vi "Handle low Press.vi"(8 "error in (no error)":errorcluster, 11 "Stand in":refnum<class "Stand.lvclass">) -> (0 "error out":errorcluster, 3 "Stand out":refnum<class "Stand.lvclass">)   [LabVIEW 2019, in "Stand.lvclass"]
uses:
  Stand.lvclass
  D:/GIT H4000/H4000/src/Device_class/Device.lvclass
  Stand.lvclass/Stand.ctl
  TypeDef/handleModeState.ctl
  Device_class/Device.lvclass/Device.ctl
  FPGA/TypeDef/DO index.ctl
  TypeDef/Active Motor.ctl
  TypeDef/Motor N.ctl
  AI_class/AI.lvclass/AI.ctl
  AnalogComparator_class/AnalogComparator.lvclass/AnalogComparator.ctl
  OscillationClass/OscillationDetector.lvclass/OscillationDetector.ctl
  AI_class/Get_Values.vi
  AnalogComparator_class/GetStatus.vi
  OscillationClass/Read DATA.vi
  FPGA_API_class/FPGA API.lvclass
  Device_class/Device.lvclass
  PM_Group_class/PM_Group.lvclass
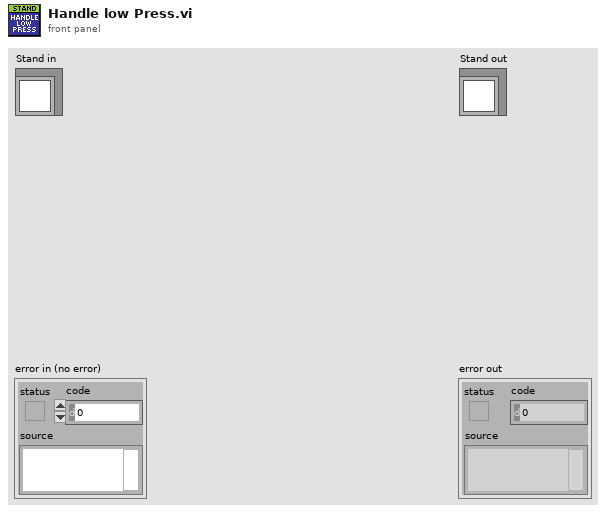
[diagram p1: front panel]
types:
  T1 = typedef "Step_Name.ctl" = enum16{"IDLE", "Filling", "Low Pressure", "Hi Pressure", "Abrupt Pressure Release", "Smooth Pressure Release", "Measuring Leakage Sensor 41.3", "Measuring Leakage Burette 42", "Alarm", "Stop Pump"}
  T2 = typedef "handleModeState.ctl" = enum16{"Init", "Run"}
  T3 = typedef "Active Motor.ctl" = cluster{"Active":bool, "MotorN":T4}
  T4 = typedef "Motor N.ctl" = enum16{"M12", "M21", "M24"}
  T5 = typedef "Direction.ctl" = enum16{"None", "DUT", "Chamber"}
  T6 = typedef "DO index.ctl" = u8
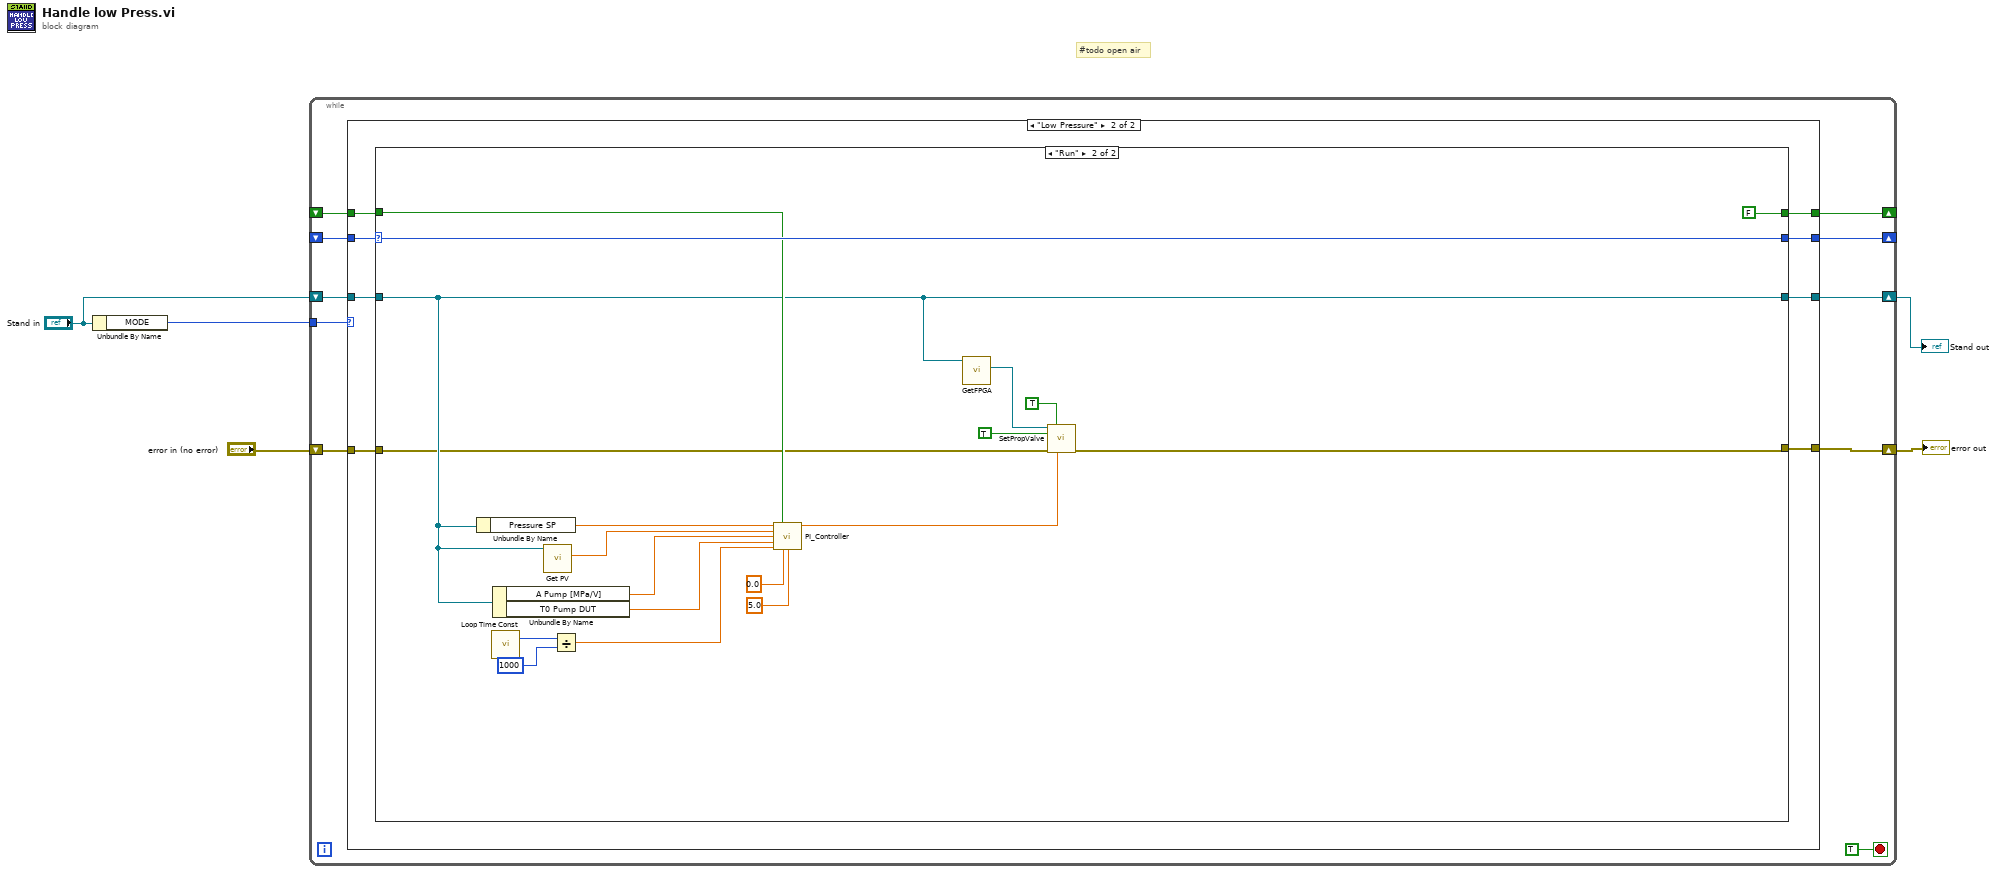
[diagram p0: block diagram]
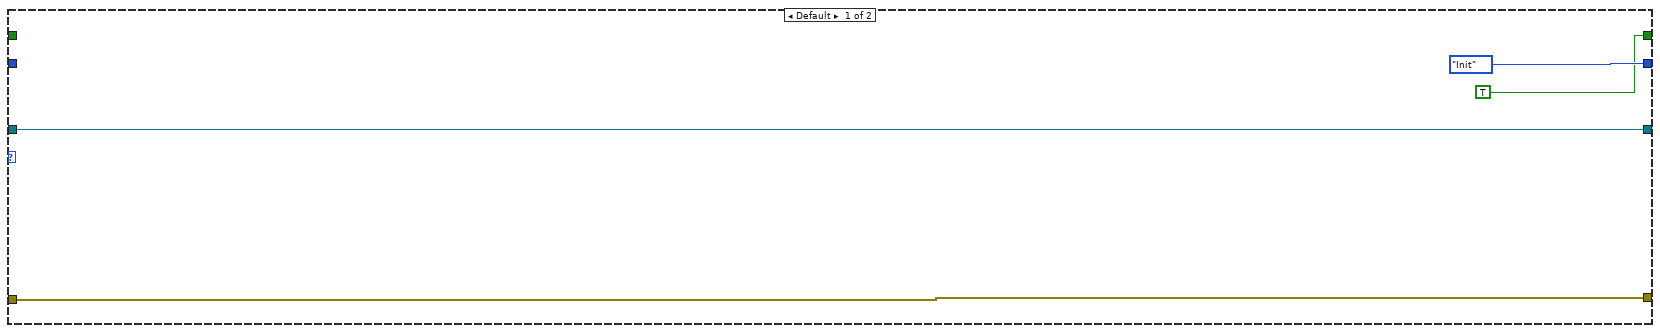
[diagram p2: hidden frame]
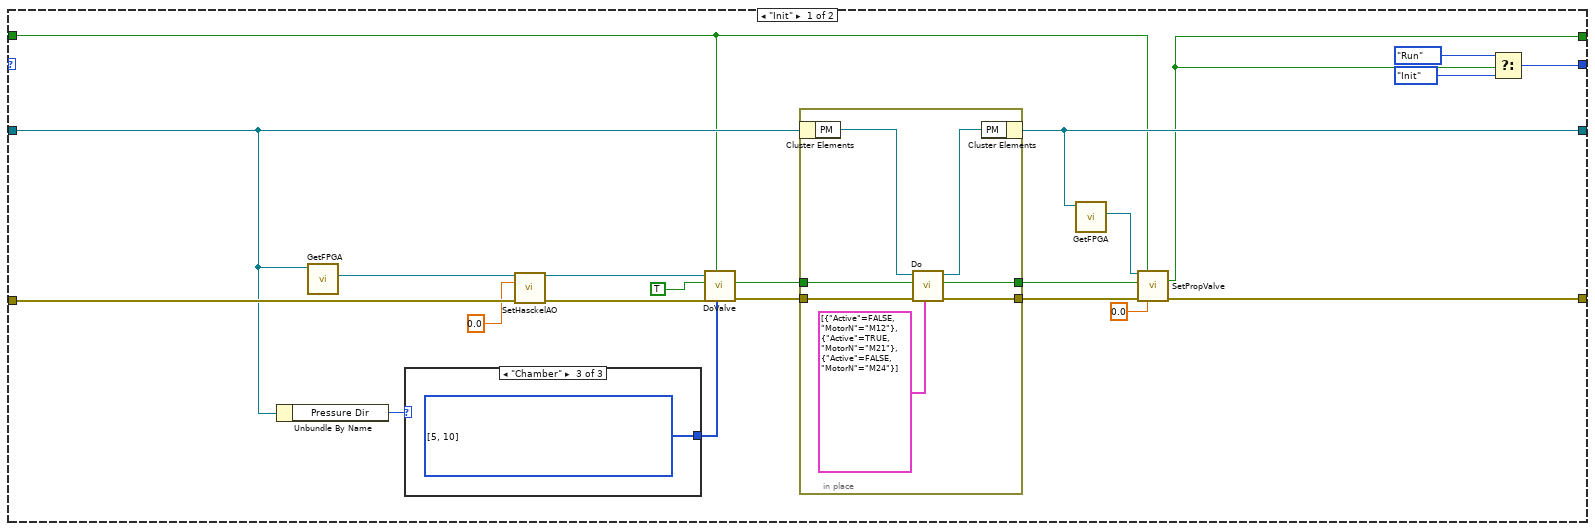
[diagram p3: hidden frame]
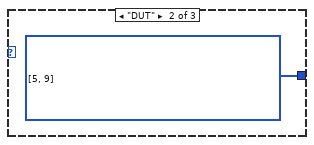
[diagram p5: hidden frame]
diagram:
  # "#todo open air"
  n1 = Unbundle By Name("Stand in") -> ("MODE"=w2:T1)
  n2 = while {
    tunnel: w2 -> [w12]
    shift-right: [w15] -> w5
    shift-left: "error in (no error)" -> [w14]
    shift-right: [w11] -> w1
    shift-left: "Stand in" -> [w13]
    shift-right: [w9] -> _
    shift-left: _ -> [w8]
    shift-right: [w7] -> _
    shift-left: _ -> [w6]
    stop <- TRUE stop-if-true
    n3 = case shown="\"Low Pressure\"" w12 {
      tunnel: w14 -> [w19 w26]
      tunnel: [w19 w27] -> w15
      tunnel: w13 -> [w18 w25]
      tunnel: [w18 w24] -> w11
      tunnel: [handleModeState."Init" ("handleModeState") w20] -> w9
      tunnel: w8 -> [_ w23]
      tunnel: [TRUE w21] -> w7
      tunnel: w6 -> [_ w22]
      frame Default {
      }
      frame "Low Pressure" {
        n4 = case shown="\"Run\"" w23 {
          selector: w23 -> [_ w77]
          tunnel: [w42 w59] -> w27
          tunnel: w26 -> [w49 w62]
          tunnel: w25 -> [w45 w64]
          tunnel: [w48 w64] -> w24
          tunnel: w22 -> [w44 w75]
          tunnel: [w28 FALSE] -> w21
          tunnel: [w47 w77] -> w20
          frame "Init" {
            n5 = Unbundle By Name(w45) -> ("Pressure Dir"=w39:T5)
            n6 = call "GetFPGA.vi"("Device in"=w45) -> ("FPGA API.lvclass"=w36:refnum<class "FPGA API.lvclass">)  [unwired: 10 in]
            n7 = case shown="\"Chamber\"" w39 {
              tunnel: [_ w50 w51] -> w38
              frame Default {
              }
              frame "DUT" {
                w50 = T6[] [5, 9] items=["DO 0 [KP1] [M12]", "DO 1 [ON KP2] [M21]", "DO 2 [ON KP3] [M24]", "DO 3 [WATER Y18.1 [DO3]]", "DO 4 [WATER Y18.2 [DO4]]", "DO 5 [KP6 Y29.1 33.7]", "DO 6 [KP7 Y29.2 33.8]", "DO 7 [KP8 Y29.3 33.9]", "DO 8 [KP9 Y29.4  33.12]", "DO 9 [KP10 Y29.5 33.1]", "DO 10 [KP11 Y29.6 33.2]", "DO 11 [KP12 Y29.7  33.13]", "DO 12 [KP13 Y29.8  33.11]", "DO 13 [KP14 Y29.9 33.10]", "DO 14 [KP15 Y29.10  33.6]", "DO 15 [KP16 Y29.11  33.5]", "DO 16 [KP17 Y29.12  33.4]", "DO 17 [KP18 Y29.13 33.3]", "DO 18 [AIR KP19]", "DO 19 [STEP DRIVE EN KP20]", "DO 20 [KP21 Y44.1 OPEN]", "DO 21 [ KP22 Y44.1 CLOSE]", "DO 22 [ KP23 Y44.2 OPEN]", "DO 23", "DO 24 [STEP DRIVE 1]", "DO 25 [STEP DRIVE 2]"] ("#DO")
              }
              frame "Chamber" {
                w51 = T6[] [5, 10] items=["DO 0 [KP1] [M12]", "DO 1 [ON KP2] [M21]", "DO 2 [ON KP3] [M24]", "DO 3 [WATER Y18.1 [DO3]]", "DO 4 [WATER Y18.2 [DO4]]", "DO 5 [KP6 Y29.1 33.7]", "DO 6 [KP7 Y29.2 33.8]", "DO 7 [KP8 Y29.3 33.9]", "DO 8 [KP9 Y29.4  33.12]", "DO 9 [KP10 Y29.5 33.1]", "DO 10 [KP11 Y29.6 33.2]", "DO 11 [KP12 Y29.7  33.13]", "DO 12 [KP13 Y29.8  33.11]", "DO 13 [KP14 Y29.9 33.10]", "DO 14 [KP15 Y29.10  33.6]", "DO 15 [KP16 Y29.11  33.5]", "DO 16 [KP17 Y29.12  33.4]", "DO 17 [KP18 Y29.13 33.3]", "DO 18 [AIR KP19]", "DO 19 [STEP DRIVE EN KP20]", "DO 20 [KP21 Y44.1 OPEN]", "DO 21 [ KP22 Y44.1 CLOSE]", "DO 22 [ KP23 Y44.2 OPEN]", "DO 23", "DO 24 [STEP DRIVE 1]", "DO 25 [STEP DRIVE 2]"] ("#DO")
              }
            }
            n8 = call-dynamic "SetHasckelAO.vi"("FPGA API in"=w36, "Haskel in"=0.0, "error in (no error)"=w49) -> ("FPGA API out"=w41:refnum<class "FPGA API.lvclass">, "error out"=w40:errorcluster)  [unwired: 11 in]
            n9 = call "DoValve.vi"("#DO"=w38, "Init"=w44, "error in (no error)"=w40, "Do"=TRUE, "reference in"=w41) -> ("error out"=w34:errorcluster, "Done"=w33:bool)  [unwired: 4 in, 1 out]
            n10 = in-place {
              in-place-border: w34 -> [w57]
              in-place-border: w33 -> [w55]
              in-place-border: [w54] -> w32
              in-place-border: [w53] -> w30
              n11 = in-place-cluster #1(w45) -> ("PM"=w58:refnum<class "PM_Group.lvclass">)
              n12 = call "Do.vi"("Data"=T3[] [{"Active"=FALSE, "MotorN"=enum."M12"}, {"Active"=TRUE, "MotorN"=enum."M21"}, {"Active"=FALSE, "MotorN"=enum."M24"}] ("Array"), "error in (no error)"=w57, "Do"=w55, "PM_Group in"=w58) -> ("error out"=w54:errorcluster, "Done"=w53:bool, "PM_Group out"=w56:refnum<class "PM_Group.lvclass">)  [unwired: 5 in]
              n13 = in-place-cluster #1("PM"=w56) -> (w48:refnum<class "Stand.lvclass">)
            }
            n14 = call "GetFPGA.vi"("Device in"=w48) -> ("FPGA API.lvclass"=w31:refnum<class "FPGA API.lvclass">)  [unwired: 10 in]
            n15 = call-dynamic "SetPropValve.vi"("FPGA API in"=w31, "Init"=w44, "Do"=w30, "error in (no error)"=w32, "AO 1"=0.0) -> ("Done"=w28:bool, "error out"=w42:errorcluster)  [unwired: 8 in, 1 out]
            n16 = Select(t=handleModeState."Run", s=w28, f=handleModeState."Init") -> (s? t:f=w47:T2)
          }
          frame "Run" {
            n17 = Unbundle By Name(w64) -> ("Pressure SP"=w74:dbl)
            n18 = call "Loop Time Const.vi"() -> ("loop time ms"=w68:i64)  [unwired: 3 in]
            n19 = Unbundle By Name(w64) -> ("A Pump [MPa/V]"=w72:dbl, "T0 Pump DUT"=w69:dbl)
            n20 = call "Get PV.vi"("Stand in"=w64) -> ("Stat Data.scl mean"=w73:dbl)  [unwired: 10 in]
            n21 = Divide(x=w68, y=i64 1000) -> (x/y=w66:dbl)
            n22 = call "PI_Controller.vi"("SP"=w74, "Init"=w75, "PV"=w73, "A"=w72, "T0"=w69, "dt"=w66, "U min"=0.0, "U max"=5.0) -> ("U out"=w63:dbl)  [unwired: 7 in]
            n23 = call "GetFPGA.vi"("Device in"=w64) -> ("FPGA API.lvclass"=w65:refnum<class "FPGA API.lvclass">)  [unwired: 10 in]
            n24 = call-dynamic "SetPropValve.vi"("FPGA API in"=w65, "Init"=TRUE, "Do"=TRUE, "error in (no error)"=w62, "AO 1"=w63) -> ("error out"=w59:errorcluster)  [unwired: 8 in, 2 out]
          }
        }
      }
    }
  }
  "error out" <- w5
  "Stand out" <- w1
